vi "VISA Channel Check.vi"(10 "VISA Channel Array":refnum<visa-resource-name>[](array[refnum])) -> (2 "Array":bool[](array[boolean]))   [LabVIEW 2012]
panel:
  out "index of element":i32
  out "find list":string[](array[string])
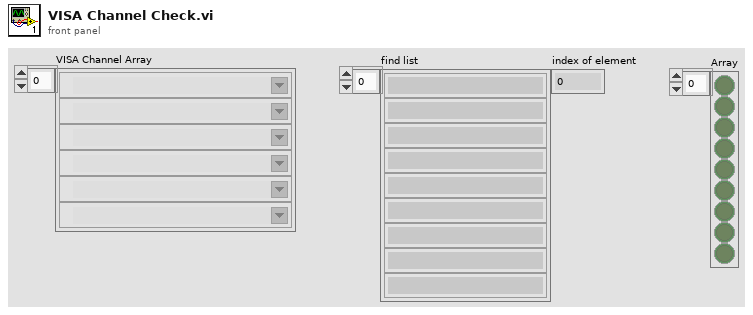
[diagram p1: front panel]
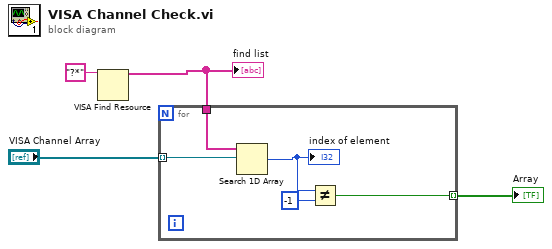
[diagram p0: block diagram]
diagram:
  n1 = VISA Find Resource(11:"?*" ("expression (\"?*\")")) -> (3:w3:string[])  [unwired: 2 in, 2 out]
  "find list" <- w3
  n2 = for {
    tunnel: w3 -> [w9]
    tunnel: [w6] -> w2 mode=indexing
    tunnel: "VISA Channel Array" -> [w5] mode=indexing
    n3 = Search 1D Array(1D array=w9, element=w5) -> (index of element=w8:i32)  [unwired: 1 in]
    "index of element" <- w8
    n4 = Not Equal?(x=w8, y=-1) -> (x != y?=w6:bool)
  }
  "Array" <- w2
